vi "T3AWG Test Panel.vi"(8 "error in (no error)":errorcluster, 11 "t3awg":T1={"VISA"="", "use ext ref"=FALSE, "ext ref [Hz]"=0.0, "load Z"=enum."High Z", "ramdac max n"=0, "noise dither [V]"=0.0, "t3awg fs rules"=[], "channels"=0, "ramdac min n"=0, "channel list"=[], "gen resl [Vpp]"=0.0, "wave data format"=enum."Binary"} {"t3awg fs rules"."fs-step [Hz]" format="%#_6p"; "t3awg fs rules"."fs-max [Hz]" format="%#_6p"; "t3awg fs rules"."for f0 <" format="%#_6p"; "t3awg fs rules"."fs-min [Hz]" format="%#_6p"}) -> (0 "error out":errorcluster, 3 "t3awg out":T1={"VISA"="", "use ext ref"=FALSE, "ext ref [Hz]"=0.0, "load Z"=enum."High Z", "ramdac max n"=0, "noise dither [V]"=0.0, "t3awg fs rules"=[], "channels"=0, "ramdac min n"=0, "channel list"=[], "gen resl [Vpp]"=0.0, "wave data format"=enum."Binary"} {"t3awg fs rules"."fs-step [Hz]" format="%#_6p"; "t3awg fs rules"."fs-max [Hz]" format="%#_6p"; "t3awg fs rules"."for f0 <" format="%#_6p"; "t3awg fs rules"."fs-min [Hz]" format="%#_6p"})   [LabVIEW 2020, in "Active Technologies AWG3000.lvlib"]
uses:
  Active Technologies AWG3000.lvlib
  T3AWG Voltage Unit.ctl
  T3AWG Session.ctl
  T3AWG Load Z.ctl
  fgen_ramdac_fs_rules.ctl
  T3AWG Channel.ctl
panel:
  out "Real freq [Hz]":dbl format="%_8p"
  out "IDN string":string
  in  "btn exit":bool
  in  "btn update":bool
  out "RAMDAC samples":i32
  out "Freq error [ppm]":dbl format="%#_6f"
  in  "Voltage unit":T6
  in  "Override default dither noise":bool
  in  "btn clear":bool
  in  "Frequency [Hz]":dbl format="%_8p"
  in  "Channels":T7(array[cluster]) {"Noise [V]" format="%#_6p"; "Amplitude [V]" format="%#_6p"}
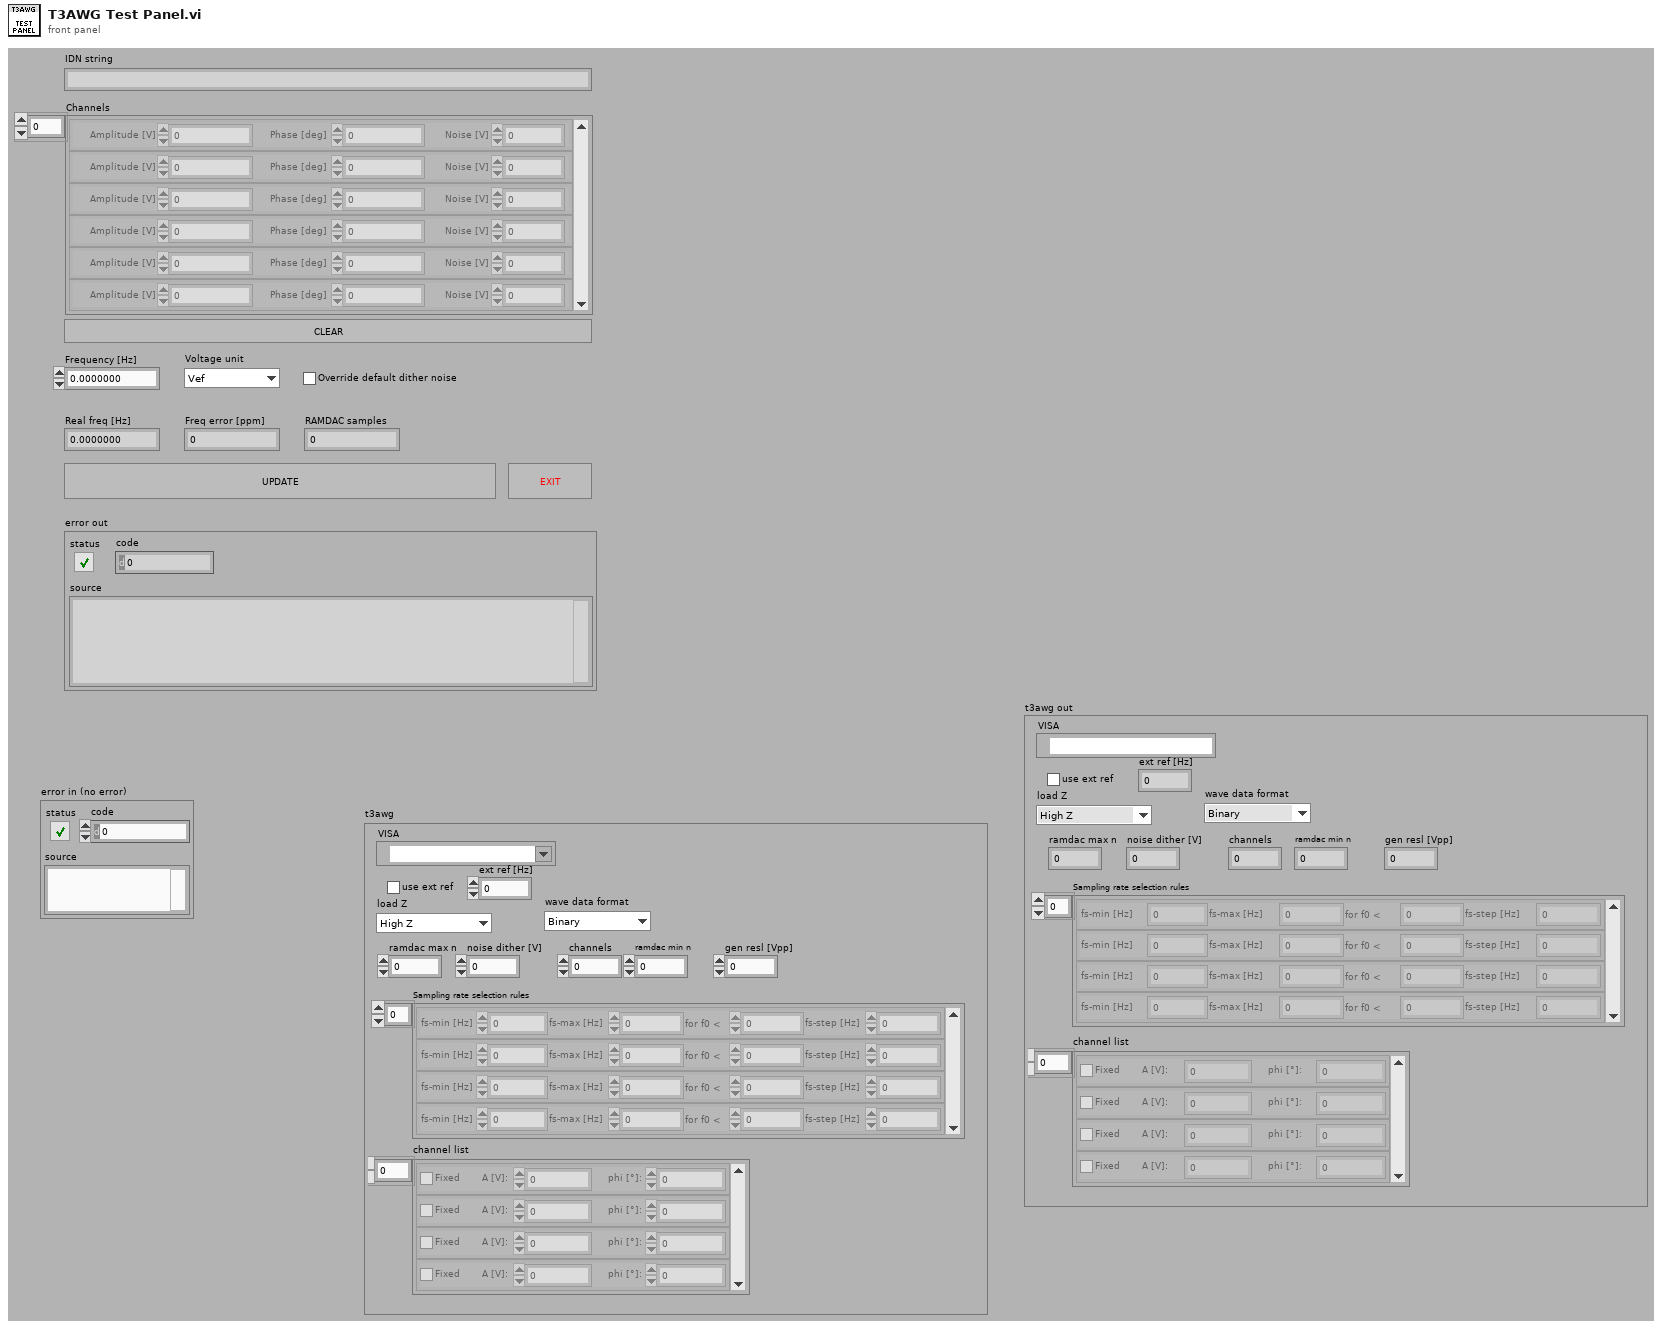
[diagram p1: front panel]
types:
  T1 = typedef "Active Technologies AWG3000.lvlib/T3AWG Session.ctl" = cluster{"VISA":refnum<visa-resource-name>, "use ext ref":bool, "ext ref [Hz]":dbl, "load Z":T2, "ramdac max n":i32, "noise dither [V]":dbl, "t3awg fs rules":T3[], "channels":i32, "ramdac min n":i32, "channel list":T4[], "gen resl [Vpp]":dbl, "wave data format":T5}
  T2 = typedef "Active Technologies AWG3000.lvlib/T3AWG Load Z.ctl" = enum16{"High Z", "50 Ohm"}
  T3 = typedef "Active Technologies AWG3000.lvlib/fgen_ramdac_fs_rules.ctl" = cluster{"fs-min [Hz]":dbl, "fs-max [Hz]":dbl, "for f0 < ":dbl, "fs-step [Hz]":dbl}
  T4 = typedef "Active Technologies AWG3000.lvlib/T3AWG Channel.ctl" = cluster{"Fixed":bool, "A [V]:":dbl, "phi [°]:":dbl}
  T5 = typedef "Active Technologies AWG3000.lvlib/T3AWG Wave Format" = enum16{"Text", "Binary"}
  T6 = typedef "Active Technologies AWG3000.lvlib/T3AWG Voltage Unit.ctl" = enum16{"Vef", "Vp", "Vpp"}
  T7 = cluster{"Amplitude [V]":dbl, "Phase [deg]":dbl, "Noise [V]":dbl}[]
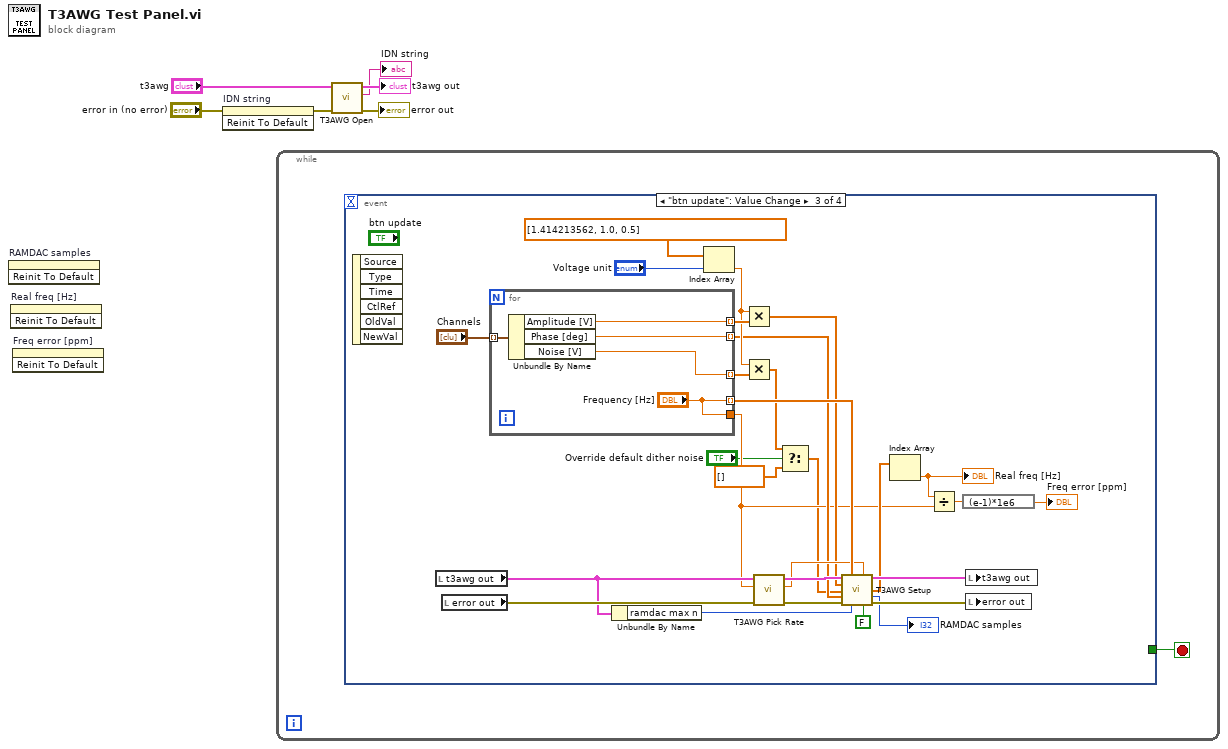
[diagram p0: block diagram]
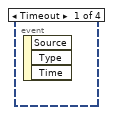
[diagram p2: hidden frame]
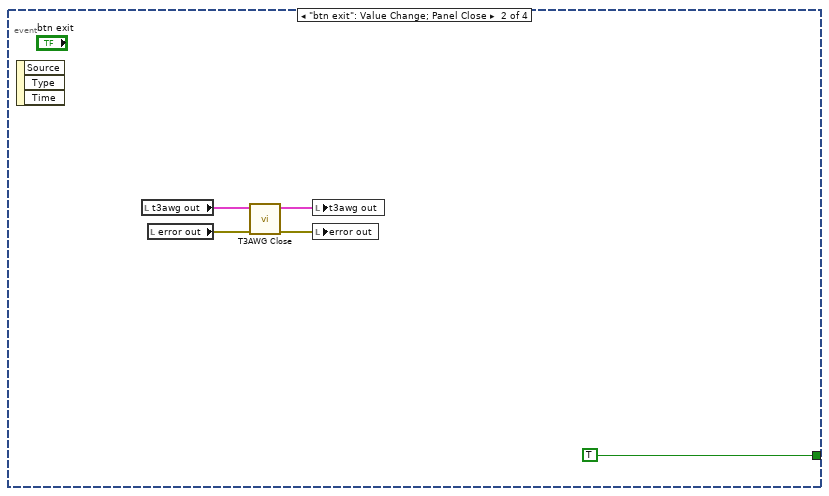
[diagram p3: hidden frame]
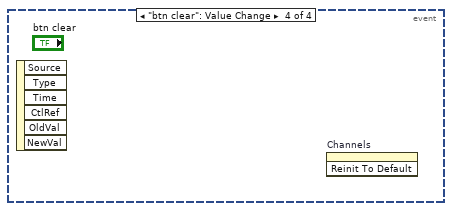
[diagram p4: hidden frame]
diagram:
  n1 = invoke on="RAMDAC samples" class="DigNum (strict)" method="Reinit To Default"() -> ()  [unwired: 3 in, 3 out]
  n2 = invoke on="Real freq [Hz]" class="DigNum (strict)" method="Reinit To Default"() -> ()  [unwired: 3 in, 3 out]
  n3 = invoke on="Freq error [ppm]" class="DigNum (strict)" method="Reinit To Default"() -> ()  [unwired: 3 in, 3 out]
  n4 = invoke on="IDN string" class="Str" method="Reinit To Default"(error in="error in (no error)") -> (error out=w1:errorcluster)  [unwired: 2 in, 2 out]
  n5 = while {
    stop <- w7 stop-if-true
    n6 = event shown="[2] \"btn update\": Value Change" {
      selector: _ -> [_ _ _ _]
      dyn-events: _ -> [_ _ _ _]
      timeout: _ -> [_ _ _ _]
      tunnel: [_ TRUE _ _] -> w7
      event Timeout {
        n7 = event-data() -> ()  [unwired: 1 in, 3 out]
      }
      event "btn exit": Value Change; Panel Close {
        n8 = event-data() -> ()  [unwired: 1 in, 3 out]
        n9 = local read "t3awg out"() -> (w11:T1)
        n10 = local read "error out"() -> (w10:errorcluster)
        n11 = call "T3AWG Close.vi"("error in (no error)"=w10, "t3awg"=w11) -> ("error out"=w8:errorcluster, "t3awg out"=w9:T1)  [unwired: 8 in]
        n12 = local write "t3awg out"(w9) -> ()
        n13 = local write "error out"(w8) -> ()
      }
      event "btn update": Value Change {
        n14 = event-data() -> ()  [unwired: 1 in, 6 out]
        n15 = local read "t3awg out"() -> (w27:T1)
        n16 = local read "error out"() -> (w28:errorcluster)
        n17 = for {
          tunnel: "Channels" -> [w45] mode=indexing
          tunnel: [w44] -> w35 mode=indexing
          tunnel: [w43] -> w23 mode=indexing
          tunnel: [w41] -> w34 mode=indexing
          tunnel: ["Frequency [Hz]"] -> w30 mode=indexing
          tunnel: ["Frequency [Hz]"] -> w21
          n18 = Unbundle By Name(w45) -> ("Amplitude [V]"=w44:dbl, "Phase [deg]"=w43:dbl, "Noise [V]"=w41:dbl)
        }
        n19 = Unbundle By Name(w27) -> ("ramdac max n"=w31:i32)
        n20 = Index Array(array=dbl[] [1.414213562, 1.0, 0.5], index="Voltage unit") -> (element=w33:dbl)
        n21 = Multiply(x=w33, y=w35) -> (x*y=w24:dbl[])
        n22 = Multiply(x=w33, y=w34) -> (x*y=w15:dbl[])
        n23 = call "T3AWG Pick Rate.vi"("error in (no error)"=w28, "f0 [Hz]"=w21, "t3awg"=w27) -> ("error out"=w29:errorcluster, "fs-min [Hz]"=w25:dbl, "t3awg out"=w26:T1)  [unwired: 6 in]
        n24 = Select(t=w15, s="Override default dither noise", f=dbl[] []) -> (s? t:f=w14:dbl[])
        n25 = call "T3AWG Setup.vi"("t3awg"=w26, "f [Hz]"=w30, "fs [Hz]"=w25, "A [-]"=w24, "noise [-]"=w14, "phi [deg]"=w23, "error in (no error)"=w29, "N"=w31, "exact setup (True)"=FALSE) -> ("t3awg out"=w39:T1, "f real [Hz]"=w22:dbl[], "RAMDAC N"=→"RAMDAC samples":i32, "error out"=w40:errorcluster)  [unwired: 3 in]
        n26 = Index Array(array=w22) -> (element=w18:dbl)  [unwired: 1 in]
        "Real freq [Hz]" <- w18
        n27 = Divide(x=w18, y=w21) -> (x/y=w20:dbl)
        n28 = expression code="(e-1)*1e6"(w20) -> (→"Freq error [ppm]":dbl)
        n29 = local write "t3awg out"(w39) -> ()
        n30 = local write "error out"(w40) -> ()
      }
      event "btn clear": Value Change {
        n31 = event-data() -> ()  [unwired: 1 in, 6 out]
        n32 = invoke on="Channels" class="Arr (strict)" method="Reinit To Default"() -> ()  [unwired: 3 in, 3 out]
      }
    }
  }
  n33 = call "T3AWG Open.vi"("error in (no error)"=w1, "t3awg"="t3awg") -> ("error out"=→"error out":errorcluster, "idn string"=→"IDN string":string, "t3awg out"=→"t3awg out":T1)  [unwired: 7 in]
